vi "Tag Names.vi"(11 "Process Name":string) -> (2 "Scale Tags":T1, 4 "All Boolean Tags":string[](array[string]), 5 "All  Numeric Tags":string[](array[string]))   [LabVIEW 2021, in "Scale Module.lvlib" / "Scale Module Engine.lvlib"]
uses:
  Scale Module Engine.lvlib
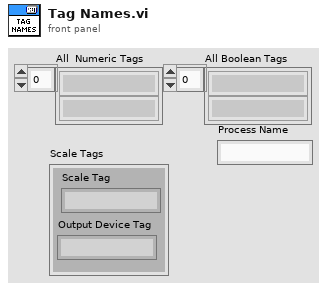
[diagram p1: front panel]
types:
  T1 = cluster{"Scale Tag":string, "Output Device Tag":string}
  T2 = cluster{"Scale Value":string, "Scale Error":string}
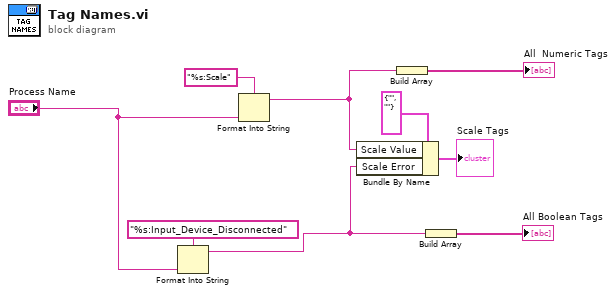
[diagram p0: block diagram]
diagram:
  n1 = Format Into String(format string="%s:Input_Device_Disconnected", "Process Name") -> (resulting string=w1:string)  [unwired: 2 in, 1 out]
  n2 = Format Into String(format string="%s:Scale", "Process Name") -> (resulting string=w3:string)  [unwired: 2 in, 1 out]
  n3 = Bundle By Name(cluster=T2 {"Scale Value"="", "Scale Error"=""} ("Scale Tags 2"), "Scale Value"=w3, "Scale Error"=w1) -> (→"Scale Tags":T2)
  n4 = Build Array(w3) -> (→"All  Numeric Tags":string[])
  n5 = Build Array(w1) -> (→"All Boolean Tags":string[])
